vi "Write Message Stream.vi"(10 "Message Stream.lvclass":refnum<class "Message Stream.lvclass">, 11 "Target Reply Time Test Actor in":refnum<class "Target Reply Time Test Actor.lvclass">) -> (3 "Target Reply Time Test Actor out":refnum<class "Target Reply Time Test Actor.lvclass">)   [LabVIEW 2023, in "Target Reply Time Test Actor.lvlib" / "Target Reply Time Test Actor.lvclass"]
uses:
  Target Reply Time Test Actor.lvclass
  <vilib>/ni/Actors/Network Endpoint Actors/Abstract Classes/Message Stream/Message Stream.lvclass
  Target Reply Time Test Actor.lvclass/Target Reply Time Test Actor.ctl
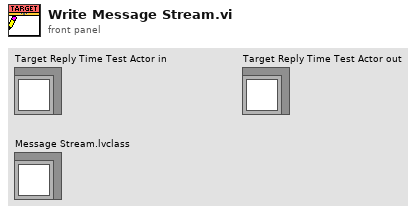
[diagram p1: front panel]
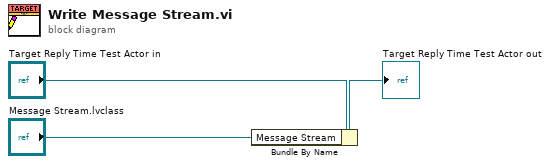
[diagram p0: block diagram]
diagram:
  n1 = Bundle By Name(cluster="Target Reply Time Test Actor in", "Message Stream"="Message Stream.lvclass") -> (→"Target Reply Time Test Actor out":refnum<class "Target Reply Time Test Actor.lvclass">)
